vi "S4GUI_002.vi"(7 "Tab ObsEng":enum32{"Obs", "CCD modes", "Eng"}(tab)) -> ()   [LabVIEW 2018] (continued)
            n2632 = call-dynamic "Write PREV_FT.vi"("error in (no error)"=w5539, "PREV_FT"=w5550, "Interface in"=w5546) -> ("error out"=w5542:errorcluster, "Interface out"=w5544:refnum<class "Interface.lvclass">)  [unwired: 7 in]
            n2633 = property on="Exptime ch3" class="DigNum (strict)"("Value"=w5707) -> ()  [unwired: 2 in, 2 out]
            n2634 = call-dynamic "Write PREV_FT.vi"("error in (no error)"=w5643, "PREV_FT"=w5656, "Interface in"=w5645) -> ("error out"=w5649:errorcluster, "Interface out"=w5642:refnum<class "Interface.lvclass">)  [unwired: 7 in]
            n2635 = call-dynamic "Write target cluster.vi"("error in (no error)"=w5591, "target cluster"=w5592, "Channel in"=w5589) -> ("error out"=w5590:errorcluster, "Channel out"=w5588:refnum<class "Channel.lvclass">)  [unwired: 7 in]
            n2636 = call-dynamic "Write target cluster.vi"("error in (no error)"=w5489, "target cluster"=w5488, "Channel in"=w5493) -> ("error out"=w5487:errorcluster, "Channel out"=w5486:refnum<class "Channel.lvclass">)  [unwired: 7 in]
            n2637 = call-dynamic "Write target cluster.vi"("error in (no error)"=w5542, "target cluster"=w5543, "Channel in"=w5537) -> ("error out"=w5538:errorcluster, "Channel out"=w5536:refnum<class "Channel.lvclass">)  [unwired: 7 in]
            n2638 = call-dynamic "Write target cluster.vi"("error in (no error)"=w5649, "target cluster"=w5652, "Channel in"=w5647) -> ("error out"=w5651:errorcluster, "Channel out"=w5650:refnum<class "Channel.lvclass">)  [unwired: 7 in]
            n2639 = Flatten To String(anything=w5592, error in (no error)=w5590) -> (data string=w5625:string, error out=w5626:errorcluster)  [unwired: 2 in, 1 out]
            n2640 = Flatten To String(anything=w5488, error in (no error)=w5487) -> (data string=w5531:string, error out=w5530:errorcluster)  [unwired: 2 in, 1 out]
            n2641 = Flatten To String(anything=w5543, error in (no error)=w5538) -> (data string=w5574:string, error out=w5575:errorcluster)  [unwired: 2 in, 1 out]
            n2642 = Flatten To String(anything=w5652, error in (no error)=w5651) -> (data string=w5684:string, error out=w5683:errorcluster)  [unwired: 2 in, 1 out]
            n2643 = property on="Exptime ch4" class="DigNum (strict)"("Value"=w5707) -> ()  [unwired: 2 in, 2 out]
            n2644 = call "Write flatted cluster.vi"("error in (no error)"=w5626, "flatted cluster"=w5625, "Interface in"=w5587) -> ("error out"=w5628:errorcluster, "Interface out"=w5627:refnum<class "Interface.lvclass">)  [unwired: 7 in]
            n2645 = call "Write flatted cluster.vi"("error in (no error)"=w5530, "flatted cluster"=w5531, "Interface in"=w5495) -> ("error out"=w5528:errorcluster, "Interface out"=w5529:refnum<class "Interface.lvclass">)  [unwired: 7 in]
            n2646 = call "Write flatted cluster.vi"("error in (no error)"=w5575, "flatted cluster"=w5574, "Interface in"=w5544) -> ("error out"=w5577:errorcluster, "Interface out"=w5576:refnum<class "Interface.lvclass">)  [unwired: 7 in]
            n2647 = call "Write flatted cluster.vi"("error in (no error)"=w5683, "flatted cluster"=w5684, "Interface in"=w5642) -> ("error out"=w5681:errorcluster, "Interface out"=w5682:refnum<class "Interface.lvclass">)  [unwired: 7 in]
            n2648 = call-dynamic "Write Interface.vi"("error in (no error)"=w5628, "Interface.lvclass"=w5627, "Channel in"=w5588) -> ("error out"=w5630:errorcluster, "Channel out"=w5631:refnum<class "Channel.lvclass">)  [unwired: 7 in]
            n2649 = call-dynamic "Write Interface.vi"("error in (no error)"=w5528, "Interface.lvclass"=w5529, "Channel in"=w5486) -> ("error out"=w5526:errorcluster, "Channel out"=w5525:refnum<class "Channel.lvclass">)  [unwired: 7 in]
            n2650 = call-dynamic "Write Interface.vi"("error in (no error)"=w5577, "Interface.lvclass"=w5576, "Channel in"=w5536) -> ("error out"=w5579:errorcluster, "Channel out"=w5580:refnum<class "Channel.lvclass">)  [unwired: 7 in]
            n2651 = call-dynamic "Write Interface.vi"("error in (no error)"=w5681, "Interface.lvclass"=w5682, "Channel in"=w5650) -> ("error out"=w5679:errorcluster, "Channel out"=w5678:refnum<class "Channel.lvclass">)  [unwired: 7 in]
            n2652 = call "Write section_name.vi"("error in (no error)"=w5630, "section_name"="CCD_ACS2", "Channel in"=w5631) -> ("error out"=w5629:errorcluster, "Channel out"=w5634:refnum<class "Channel.lvclass">)  [unwired: 7 in]
            n2653 = call "Write section_name.vi"("error in (no error)"=w5526, "section_name"="CCD_ACS4", "Channel in"=w5525) -> ("error out"=w5527:errorcluster, "Channel out"=w5522:refnum<class "Channel.lvclass">)  [unwired: 7 in]
            n2654 = call "Write section_name.vi"("error in (no error)"=w5579, "section_name"="CCD_ACS3", "Channel in"=w5580) -> ("error out"=w5578:errorcluster, "Channel out"=w5583:refnum<class "Channel.lvclass">)  [unwired: 7 in]
            n2655 = call "Write section_name.vi"("error in (no error)"=w5679, "section_name"="CCD_ACS1", "Channel in"=w5678) -> ("error out"=w5680:errorcluster, "Channel out"=w5675:refnum<class "Channel.lvclass">)  [unwired: 7 in]
            n2656 = call-dynamic "save config.vi"("error in (no error)"=w5629, "file config"="lastsaved.cfg", "Channel in"=w5634) -> ("error out"=w5604:errorcluster, "Channel out"=w5605:refnum<class "Channel.lvclass">)  [unwired: 7 in]
            n2657 = call-dynamic "save config.vi"("error in (no error)"=w5527, "file config"="lastsaved.cfg", "Channel in"=w5522) -> ("error out"=w5503:errorcluster, "Channel out"=w5504:refnum<class "Channel.lvclass">)  [unwired: 7 in]
            n2658 = call-dynamic "save config.vi"("error in (no error)"=w5578, "file config"="lastsaved.cfg", "Channel in"=w5583) -> ("error out"=w5552:errorcluster, "Channel out"=w5554:refnum<class "Channel.lvclass">)  [unwired: 7 in]
            n2659 = call-dynamic "save config.vi"("error in (no error)"=w5680, "file config"="lastsaved.cfg", "Channel in"=w5675) -> ("error out"=w5665:errorcluster, "Channel out"=w5666:refnum<class "Channel.lvclass">)  [unwired: 7 in]
            n2660 = local read "Filter2"() -> (w5606:u8)
            n2661 = local read "Filter4"() -> (w5520:u8)
            n2662 = local read "Filter3"() -> (w5570:u8)
            n2663 = local read "Filter1"() -> (w5667:u8)
            n2664 = call-dynamic "Write Filter.vi"("error in (no error)"=w5604, "Filter"=w5606, "Channel in"=w5605) -> ("error out"=w5613:errorcluster, "Channel out"=w5614:refnum<class "Channel.lvclass">)  [unwired: 7 in]
            n2665 = call-dynamic "Write Filter.vi"("error in (no error)"=w5503, "Filter"=w5520, "Channel in"=w5504) -> ("error out"=w5513:errorcluster, "Channel out"=w5512:refnum<class "Channel.lvclass">)  [unwired: 7 in]
            n2666 = call-dynamic "Write Filter.vi"("error in (no error)"=w5552, "Filter"=w5570, "Channel in"=w5554) -> ("error out"=w5563:errorcluster, "Channel out"=w5562:refnum<class "Channel.lvclass">)  [unwired: 7 in]
            n2667 = call-dynamic "Write Filter.vi"("error in (no error)"=w5665, "Filter"=w5667, "Channel in"=w5666) -> ("error out"=w5674:errorcluster, "Channel out"=w5664:refnum<class "Channel.lvclass">)  [unwired: 7 in]
            n2668 = call-dynamic "Read Interface.vi"("error in (no error)"=w5613, "Channel in"=w5614) -> ("error out"=w5611:errorcluster, "Interface.lvclass"=w5616:refnum<class "Interface.lvclass">, "Channel out"=w5615:refnum<class "Channel.lvclass">)  [unwired: 7 in]
            n2669 = call-dynamic "Read Interface.vi"("error in (no error)"=w5513, "Channel in"=w5512) -> ("error out"=w5515:errorcluster, "Interface.lvclass"=w5510:refnum<class "Interface.lvclass">, "Channel out"=w5511:refnum<class "Channel.lvclass">)  [unwired: 7 in]
            n2670 = call-dynamic "Read Interface.vi"("error in (no error)"=w5563, "Channel in"=w5562) -> ("error out"=w5565:errorcluster, "Interface.lvclass"=w5560:refnum<class "Interface.lvclass">, "Channel out"=w5561:refnum<class "Channel.lvclass">)  [unwired: 7 in]
            n2671 = call-dynamic "Read Interface.vi"("error in (no error)"=w5674, "Channel in"=w5664) -> ("error out"=w5672:errorcluster, "Interface.lvclass"=w5663:refnum<class "Interface.lvclass">, "Channel out"=w5657:refnum<class "Channel.lvclass">)  [unwired: 7 in]
            n2672 = call-dynamic "Write Suffix.vi"("error in (no error)"=w5611, "Suffix"=w5689, "Interface in"=w5616) -> ("error out"=w5607:errorcluster, "Interface out"=w5617:refnum<class "Interface.lvclass">)  [unwired: 7 in]
            n2673 = call-dynamic "Write Suffix.vi"("error in (no error)"=w5515, "Suffix"=w5689, "Interface in"=w5510) -> ("error out"=w5519:errorcluster, "Interface out"=w5509:refnum<class "Interface.lvclass">)  [unwired: 7 in]
            n2674 = call-dynamic "Write Suffix.vi"("error in (no error)"=w5565, "Suffix"=w5689, "Interface in"=w5560) -> ("error out"=w5569:errorcluster, "Interface out"=w5559:refnum<class "Interface.lvclass">)  [unwired: 7 in]
            n2675 = call-dynamic "Write Suffix.vi"("error in (no error)"=w5672, "Suffix"=w5689, "Interface in"=w5663) -> ("error out"=w5668:errorcluster, "Interface out"=w5662:refnum<class "Interface.lvclass">)  [unwired: 7 in]
            n2676 = call-dynamic "Write ObsType.vi"("error in (no error)"=w5607, "ObsType"=w5688, "Interface in"=w5617) -> ("error out"=w5608:errorcluster, "Interface out"=w5618:refnum<class "Interface.lvclass">)  [unwired: 7 in]
            n2677 = call-dynamic "Write ObsType.vi"("error in (no error)"=w5519, "ObsType"=w5688, "Interface in"=w5509) -> ("error out"=w5518:errorcluster, "Interface out"=w5508:refnum<class "Interface.lvclass">)  [unwired: 7 in]
            n2678 = call-dynamic "Write ObsType.vi"("error in (no error)"=w5569, "ObsType"=w5688, "Interface in"=w5559) -> ("error out"=w5568:errorcluster, "Interface out"=w5558:refnum<class "Interface.lvclass">)  [unwired: 7 in]
            n2679 = call-dynamic "Write ObsType.vi"("error in (no error)"=w5668, "ObsType"=w5688, "Interface in"=w5662) -> ("error out"=w5669:errorcluster, "Interface out"=w5661:refnum<class "Interface.lvclass">)  [unwired: 7 in]
            n2680 = call-dynamic "Write Object.vi"("error in (no error)"=w5608, "Object"=w5690, "Interface in"=w5618) -> ("error out"=w5609:errorcluster, "Interface out"=w5619:refnum<class "Interface.lvclass">)  [unwired: 7 in]
            n2681 = call-dynamic "Write Object.vi"("error in (no error)"=w5518, "Object"=w5690, "Interface in"=w5508) -> ("error out"=w5517:errorcluster, "Interface out"=w5507:refnum<class "Interface.lvclass">)  [unwired: 7 in]
            n2682 = call-dynamic "Write Object.vi"("error in (no error)"=w5568, "Object"=w5690, "Interface in"=w5558) -> ("error out"=w5567:errorcluster, "Interface out"=w5557:refnum<class "Interface.lvclass">)  [unwired: 7 in]
            n2683 = call-dynamic "Write Object.vi"("error in (no error)"=w5669, "Object"=w5690, "Interface in"=w5661) -> ("error out"=w5670:errorcluster, "Interface out"=w5660:refnum<class "Interface.lvclass">)  [unwired: 7 in]
            n2684 = call-dynamic "Write Comments.vi"("error in (no error)"=w5609, "Comments"=w5691, "Interface in"=w5619) -> ("error out"=w5610:errorcluster, "Interface out"=w5620:refnum<class "Interface.lvclass">)  [unwired: 7 in]
            n2685 = call-dynamic "Write Comments.vi"("error in (no error)"=w5517, "Comments"=w5691, "Interface in"=w5507) -> ("error out"=w5516:errorcluster, "Interface out"=w5506:refnum<class "Interface.lvclass">)  [unwired: 7 in]
            n2686 = call-dynamic "Write Comments.vi"("error in (no error)"=w5567, "Comments"=w5691, "Interface in"=w5557) -> ("error out"=w5566:errorcluster, "Interface out"=w5556:refnum<class "Interface.lvclass">)  [unwired: 7 in]
            n2687 = call-dynamic "Write Comments.vi"("error in (no error)"=w5670, "Comments"=w5691, "Interface in"=w5660) -> ("error out"=w5671:errorcluster, "Interface out"=w5659:refnum<class "Interface.lvclass">)  [unwired: 7 in]
            n2688 = call-dynamic "Write Observer.vi"("error in (no error)"=w5516, "Observer"=w5692, "Interface in"=w5506) -> ("error out"=w5514:errorcluster, "Interface out"=w5505:refnum<class "Interface.lvclass">)  [unwired: 7 in]
            n2689 = call-dynamic "Write Observer.vi"("error in (no error)"=w5566, "Observer"=w5692, "Interface in"=w5556) -> ("error out"=w5564:errorcluster, "Interface out"=w5555:refnum<class "Interface.lvclass">)  [unwired: 7 in]
            n2690 = call-dynamic "Write Observer.vi"("error in (no error)"=w5610, "Observer"=w5692, "Interface in"=w5620) -> ("error out"=w5612:errorcluster, "Interface out"=w5621:refnum<class "Interface.lvclass">)  [unwired: 7 in]
            n2691 = call-dynamic "Write Observer.vi"("error in (no error)"=w5671, "Observer"=w5692, "Interface in"=w5659) -> ("error out"=w5673:errorcluster, "Interface out"=w5658:refnum<class "Interface.lvclass">)  [unwired: 7 in]
            n2692 = call-dynamic "Write Interface.vi"("error in (no error)"=w5514, "Interface.lvclass"=w5505, "Channel in"=w5511) -> ("error out"=w5502:errorcluster, "Channel out"=w5501:refnum<class "Channel.lvclass">)  [unwired: 7 in]
            n2693 = call-dynamic "Write Interface.vi"("error in (no error)"=w5564, "Interface.lvclass"=w5555, "Channel in"=w5561) -> ("error out"=w5551:errorcluster, "Channel out"=w5553:refnum<class "Channel.lvclass">)  [unwired: 7 in]
            n2694 = call-dynamic "Write Interface.vi"("error in (no error)"=w5673, "Interface.lvclass"=w5658, "Channel in"=w5657) -> ("error out"=w5640:errorcluster, "Channel out"=w5641:refnum<class "Channel.lvclass">)  [unwired: 7 in]
            n2695 = call-dynamic "Write Interface.vi"("error in (no error)"=w5612, "Interface.lvclass"=w5621, "Channel in"=w5615) -> ("error out"=w5603:errorcluster, "Channel out"=w5602:refnum<class "Channel.lvclass">)  [unwired: 7 in]
            n2696 = case shown="True" w5637 {
              tunnel: w5641 -> [w5812 w5816]
              tunnel: w5640 -> [w5811 w5815]
              tunnel: [w5812 w5814] -> w5639
              tunnel: [w5811 w5813] -> w5638
              frame False {
              }
              frame True {
                n2697 = call-dynamic "Read State Machine.vi"("error in (no error)"=w5815, "Device in"=w5816) -> ("error out"=w5818:errorcluster, "State Machine.lvclass"=w5821:refnum<class "State Machine.lvclass">, "Device out"=w5833:refnum<class "Channel.lvclass">)  [unwired: 7 in]
                n2698 = call-dynamic "Read ref StatesQueue.vi"("error in (no error)"=w5818, "State Machine in"=w5821) -> ("error out"=w5825:errorcluster, "ref StatesQueue"=w5824:refnum<queue>, "State Machine out"=w5820:refnum<class "State Machine.lvclass">)  [unwired: 7 in]
                n2699 = Flush Queue(queue=w5824, error in (no error)=w5825) -> (queue out=w5826:refnum<queue>, error out=w5830:errorcluster)  [unwired: 1 out]
                n2700 = Enqueue Element(queue=w5826, element=u32 300 ("State"), error in (no error)=w5830) -> (queue out=w5827:refnum<queue>, error out=w5831:errorcluster)  [unwired: 1 in, 1 out]
                n2701 = Enqueue Element(queue=w5827, element=u32 60 ("State"), error in (no error)=w5831) -> (queue out=w5828:refnum<queue>, error out=w5829:errorcluster)  [unwired: 1 in, 1 out]
                n2702 = call-dynamic "Write ref StatesQueue.vi"("error in (no error)"=w5829, "ref StatesQueue"=w5828, "State Machine in"=w5820) -> ("error out"=w5817:errorcluster, "State Machine out"=w5819:refnum<class "State Machine.lvclass">)  [unwired: 7 in]
                n2703 = call-dynamic "Write State.vi"("error in (no error)"=w5817, "State"=0, "State Machine in"=w5819) -> ("error out"=w5835:errorcluster, "State Machine out"=w5832:refnum<class "State Machine.lvclass">)  [unwired: 7 in]
                n2704 = call-dynamic "Write State Machine.vi"("error in (no error)"=w5835, "State Machine.lvclass"=w5832, "Device in"=w5833) -> ("error out"=w5813:errorcluster, "Device out"=w5814:refnum<class "Channel.lvclass">)  [unwired: 7 in]
              }
            }
            n2705 = case shown="True" w5586 {
              tunnel: [w5780 w5804] -> w5636
              tunnel: [w5781 w5803] -> w5635
              tunnel: w5603 -> [w5780 w5798]
              tunnel: w5602 -> [w5781 w5797]
              frame False {
              }
              frame True {
                n2706 = call-dynamic "Read State Machine.vi"("error in (no error)"=w5798, "Device in"=w5797) -> ("error out"=w5783:errorcluster, "State Machine.lvclass"=w5785:refnum<class "State Machine.lvclass">, "Device out"=w5801:refnum<class "Channel.lvclass">)  [unwired: 7 in]
                n2707 = call-dynamic "Read ref StatesQueue.vi"("error in (no error)"=w5783, "State Machine in"=w5785) -> ("error out"=w5790:errorcluster, "ref StatesQueue"=w5789:refnum<queue>, "State Machine out"=w5786:refnum<class "State Machine.lvclass">)  [unwired: 7 in]
                n2708 = Flush Queue(queue=w5789, error in (no error)=w5790) -> (queue out=w5791:refnum<queue>, error out=w5795:errorcluster)  [unwired: 1 out]
                n2709 = Enqueue Element(queue=w5791, element=u32 300 ("State"), error in (no error)=w5795) -> (queue out=w5792:refnum<queue>, error out=w5796:errorcluster)  [unwired: 1 in, 1 out]
                n2710 = Enqueue Element(queue=w5792, element=u32 60 ("State"), error in (no error)=w5796) -> (queue out=w5793:refnum<queue>, error out=w5794:errorcluster)  [unwired: 1 in, 1 out]
                n2711 = call-dynamic "Write ref StatesQueue.vi"("error in (no error)"=w5794, "ref StatesQueue"=w5793, "State Machine in"=w5786) -> ("error out"=w5782:errorcluster, "State Machine out"=w5784:refnum<class "State Machine.lvclass">)  [unwired: 7 in]
                n2712 = call-dynamic "Write State.vi"("error in (no error)"=w5782, "State"=0, "State Machine in"=w5784) -> ("error out"=w5799:errorcluster, "State Machine out"=w5802:refnum<class "State Machine.lvclass">)  [unwired: 7 in]
                n2713 = call-dynamic "Write State Machine.vi"("error in (no error)"=w5799, "State Machine.lvclass"=w5802, "Device in"=w5801) -> ("error out"=w5804:errorcluster, "Device out"=w5803:refnum<class "Channel.lvclass">)  [unwired: 7 in]
              }
            }
            n2714 = case shown="True" w5535 {
              tunnel: [w5750 w5773] -> w5585
              tunnel: [w5749 w5772] -> w5584
              tunnel: w5553 -> [w5749 w5767]
              tunnel: w5551 -> [w5750 w5766]
              frame False {
              }
              frame True {
                n2715 = call-dynamic "Read State Machine.vi"("error in (no error)"=w5766, "Device in"=w5767) -> ("error out"=w5752:errorcluster, "State Machine.lvclass"=w5754:refnum<class "State Machine.lvclass">, "Device out"=w5770:refnum<class "Channel.lvclass">)  [unwired: 7 in]
                n2716 = call-dynamic "Read ref StatesQueue.vi"("error in (no error)"=w5752, "State Machine in"=w5754) -> ("error out"=w5759:errorcluster, "ref StatesQueue"=w5758:refnum<queue>, "State Machine out"=w5755:refnum<class "State Machine.lvclass">)  [unwired: 7 in]
                n2717 = Flush Queue(queue=w5758, error in (no error)=w5759) -> (queue out=w5760:refnum<queue>, error out=w5764:errorcluster)  [unwired: 1 out]
                n2718 = Enqueue Element(queue=w5760, element=u32 300 ("State"), error in (no error)=w5764) -> (queue out=w5761:refnum<queue>, error out=w5765:errorcluster)  [unwired: 1 in, 1 out]
                n2719 = Enqueue Element(queue=w5761, element=u32 60 ("State"), error in (no error)=w5765) -> (queue out=w5762:refnum<queue>, error out=w5763:errorcluster)  [unwired: 1 in, 1 out]
                n2720 = call-dynamic "Write ref StatesQueue.vi"("error in (no error)"=w5763, "ref StatesQueue"=w5762, "State Machine in"=w5755) -> ("error out"=w5751:errorcluster, "State Machine out"=w5753:refnum<class "State Machine.lvclass">)  [unwired: 7 in]
                n2721 = call-dynamic "Write State.vi"("error in (no error)"=w5751, "State"=0, "State Machine in"=w5753) -> ("error out"=w5768:errorcluster, "State Machine out"=w5771:refnum<class "State Machine.lvclass">)  [unwired: 7 in]
                n2722 = call-dynamic "Write State Machine.vi"("error in (no error)"=w5768, "State Machine.lvclass"=w5771, "Device in"=w5770) -> ("error out"=w5773:errorcluster, "Device out"=w5772:refnum<class "Channel.lvclass">)  [unwired: 7 in]
              }
            }
            n2723 = case shown="True" w5484 {
              tunnel: [w5718 w5738] -> w5521
              tunnel: w5502 -> [w5718 w5737]
              tunnel: w5501 -> [w5719 w5736]
              tunnel: [w5719 w5720] -> w5485
              frame False {
              }
              frame True {
                n2724 = call-dynamic "Read State Machine.vi"("error in (no error)"=w5737, "Device in"=w5736) -> ("error out"=w5723:errorcluster, "State Machine.lvclass"=w5724:refnum<class "State Machine.lvclass">, "Device out"=w5740:refnum<class "Channel.lvclass">)  [unwired: 7 in]
                n2725 = call-dynamic "Read ref StatesQueue.vi"("error in (no error)"=w5723, "State Machine in"=w5724) -> ("error out"=w5729:errorcluster, "ref StatesQueue"=w5728:refnum<queue>, "State Machine out"=w5725:refnum<class "State Machine.lvclass">)  [unwired: 7 in]
                n2726 = Flush Queue(queue=w5728, error in (no error)=w5729) -> (queue out=w5730:refnum<queue>, error out=w5734:errorcluster)  [unwired: 1 out]
                n2727 = Enqueue Element(queue=w5730, element=u32 300 ("State"), error in (no error)=w5734) -> (queue out=w5731:refnum<queue>, error out=w5735:errorcluster)  [unwired: 1 in, 1 out]
                n2728 = Enqueue Element(queue=w5731, element=u32 60 ("State"), error in (no error)=w5735) -> (queue out=w5732:refnum<queue>, error out=w5733:errorcluster)  [unwired: 1 in, 1 out]
                n2729 = call-dynamic "Write ref StatesQueue.vi"("error in (no error)"=w5733, "ref StatesQueue"=w5732, "State Machine in"=w5725) -> ("error out"=w5722:errorcluster, "State Machine out"=w5721:refnum<class "State Machine.lvclass">)  [unwired: 7 in]
                n2730 = call-dynamic "Write State.vi"("error in (no error)"=w5722, "State"=0, "State Machine in"=w5721) -> ("error out"=w5742:errorcluster, "State Machine out"=w5739:refnum<class "State Machine.lvclass">)  [unwired: 7 in]
                n2731 = call-dynamic "Write State Machine.vi"("error in (no error)"=w5742, "State Machine.lvclass"=w5739, "Device in"=w5740) -> ("error out"=w5738:errorcluster, "Device out"=w5720:refnum<class "Channel.lvclass">)  [unwired: 7 in]
              }
            }
            n2732 = call-dynamic "Write Channel.vi"("error in (no error)"=w5636, "Channel.lvclass"=w5635, "Acquisition in"=w5622) -> ("error out"=w5714:errorcluster, "Acquisition out"=w5715:refnum<class "Acquisition.lvclass">)  [unwired: 7 in]
            n2733 = call-dynamic "Write Channel.vi"("error in (no error)"=w5638, "Channel.lvclass"=w5639, "Acquisition in"=w5687) -> ("error out"=w5716:errorcluster, "Acquisition out"=w5717:refnum<class "Acquisition.lvclass">)  [unwired: 7 in]
            n2734 = call-dynamic "Write Channel.vi"("error in (no error)"=w5585, "Channel.lvclass"=w5584, "Acquisition in"=w5571) -> ("error out"=w5712:errorcluster, "Acquisition out"=w5713:refnum<class "Acquisition.lvclass">)  [unwired: 7 in]
            n2735 = call-dynamic "Write Channel.vi"("error in (no error)"=w5521, "Channel.lvclass"=w5485, "Acquisition in"=w5534) -> ("error out"=w5710:errorcluster, "Acquisition out"=w5711:refnum<class "Acquisition.lvclass">)  [unwired: 7 in]
          }
          frame "DARK" {
            # "nome do arquivo .cfg"
            # "seção no arquivo .cfg"
            # "closed"
            # "nome do arquivo .cfg"
            # "seção no arquivo .cfg"
            # "closed"
            # "nome do arquivo .cfg"
            # "seção no arquivo .cfg"
            # "closed"
            # "nome do arquivo .cfg"
            # "seção no arquivo .cfg"
            # "closed"
            # "DARK: Shutter automatically closed and restore FRAME_TRANSFER."
            n2736 = call "Read connection.vi"("error in (no error)"=w6063, "Server in"=w6064) -> ("error out"=w6069:errorcluster, "connection"=w5842:bool, "Server out"=w6070:refnum<class "Acquisition.lvclass">)  [unwired: 7 in]
            n2737 = call "Read connection.vi"("error in (no error)"=w6067, "Server in"=w6068) -> ("error out"=w6073:errorcluster, "connection"=w5844:bool, "Server out"=w6074:refnum<class "Acquisition.lvclass">)  [unwired: 7 in]
            n2738 = call "Read connection.vi"("error in (no error)"=w6065, "Server in"=w6066) -> ("error out"=w6071:errorcluster, "connection"=w5843:bool, "Server out"=w6072:refnum<class "Acquisition.lvclass">)  [unwired: 7 in]
            n2739 = call "Read connection.vi"("error in (no error)"=w6077, "Server in"=w6078) -> ("error out"=w6075:errorcluster, "connection"=w5845:bool, "Server out"=w6076:refnum<class "Acquisition.lvclass">)  [unwired: 7 in]
            n2740 = call-dynamic "Read Channel.vi"("error in (no error)"=w6069, "Acquisition in"=w6070) -> ("error out"=w5896:errorcluster, "Channel.lvclass"=w5897:refnum<class "Channel.lvclass">, "Acquisition out"=w5898:refnum<class "Acquisition.lvclass">)  [unwired: 7 in]
            n2741 = call-dynamic "Read Channel.vi"("error in (no error)"=w6073, "Acquisition in"=w6074) -> ("error out"=w5991:errorcluster, "Channel.lvclass"=w5990:refnum<class "Channel.lvclass">, "Acquisition out"=w5989:refnum<class "Acquisition.lvclass">)  [unwired: 7 in]
            n2742 = call-dynamic "Read Channel.vi"("error in (no error)"=w6075, "Acquisition in"=w6076) -> ("error out"=w6055:errorcluster, "Channel.lvclass"=w6056:refnum<class "Channel.lvclass">, "Acquisition out"=w6057:refnum<class "Acquisition.lvclass">)  [unwired: 7 in]
            n2743 = call-dynamic "Read Channel.vi"("error in (no error)"=w6071, "Acquisition in"=w6072) -> ("error out"=w5938:errorcluster, "Channel.lvclass"=w5937:refnum<class "Channel.lvclass">, "Acquisition out"=w5936:refnum<class "Acquisition.lvclass">)  [unwired: 7 in]
            n2744 = call-dynamic "Read Interface.vi"("error in (no error)"=w5896, "Channel in"=w5897) -> ("error out"=w5859:errorcluster, "Interface.lvclass"=w5858:refnum<class "Interface.lvclass">, "Channel out"=w5854:refnum<class "Channel.lvclass">)  [unwired: 7 in]
            n2745 = call-dynamic "Read Interface.vi"("error in (no error)"=w5991, "Channel in"=w5990) -> ("error out"=w5965:errorcluster, "Interface.lvclass"=w5964:refnum<class "Interface.lvclass">, "Channel out"=w5960:refnum<class "Channel.lvclass">)  [unwired: 7 in]
            n2746 = call-dynamic "Read Interface.vi"("error in (no error)"=w6055, "Channel in"=w6056) -> ("error out"=w6017:errorcluster, "Interface.lvclass"=w6018:refnum<class "Interface.lvclass">, "Channel out"=w6013:refnum<class "Channel.lvclass">)  [unwired: 7 in]
            n2747 = call-dynamic "Read Interface.vi"("error in (no error)"=w5938, "Channel in"=w5937) -> ("error out"=w5910:errorcluster, "Interface.lvclass"=w5912:refnum<class "Interface.lvclass">, "Channel out"=w5907:refnum<class "Channel.lvclass">)  [unwired: 7 in]
            n2748 = call-dynamic "Read restoreExpTime.vi"("error in (no error)"=w5965, "Interface in"=w5964) -> ("error out"=w5962:errorcluster, "restoreExpTime"=w5961:bool, "Interface out"=w5963:refnum<class "Interface.lvclass">)  [unwired: 7 in]
            n2749 = call-dynamic "Read restoreExpTime.vi"("error in (no error)"=w6017, "Interface in"=w6018) -> ("error out"=w6015:errorcluster, "restoreExpTime"=w6014:bool, "Interface out"=w6016:refnum<class "Interface.lvclass">)  [unwired: 7 in]
            n2750 = call-dynamic "Read restoreExpTime.vi"("error in (no error)"=w5859, "Interface in"=w5858) -> ("error out"=w5856:errorcluster, "restoreExpTime"=w5855:bool, "Interface out"=w5857:refnum<class "Interface.lvclass">)  [unwired: 7 in]
            n2751 = call-dynamic "Read restoreExpTime.vi"("error in (no error)"=w5910, "Interface in"=w5912) -> ("error out"=w5909:errorcluster, "restoreExpTime"=w5908:bool, "Interface out"=w5911:refnum<class "Interface.lvclass">)  [unwired: 7 in]
            n2752 = case shown="True" w5961 {
              tunnel: w5963 -> [w6208 w6213]
              tunnel: [w6208 w6216] -> w5967
              tunnel: w5962 -> [w6207 w6211]
              tunnel: [w6207 w6215] -> w5966
              frame False {
              }
              frame True {
                n2753 = call-dynamic "Write restoreExpTime.vi"("error in (no error)"=w6211, "restoreExpTime"=FALSE, "Interface in"=w6213) -> ("error out"=w6210:errorcluster, "Interface out"=w6212:refnum<class "Interface.lvclass">)  [unwired: 7 in]
                n2754 = call-dynamic "Read prev ExpTime.vi"("error in (no error)"=w6210, "Interface in"=w6212) -> ("error out"=w6215:errorcluster, "prev ExpTime"=w6214:dbl, "Interface out"=w6216:refnum<class "Interface.lvclass">)  [unwired: 7 in]
                n2755 = property on="Exptime ch2" class="DigNum (strict)"("Value"=w6214) -> ()  [unwired: 2 in, 2 out]
              }
            }
            n2756 = case shown="True" w6014 {
              tunnel: [w6218 w6226] -> w6020
              tunnel: [w6217 w6225] -> w6019
              tunnel: w6016 -> [w6218 w6223]
              tunnel: w6015 -> [w6217 w6221]
              frame False {
              }
              frame True {
                n2757 = call-dynamic "Write restoreExpTime.vi"("error in (no error)"=w6221, "restoreExpTime"=FALSE, "Interface in"=w6223) -> ("error out"=w6220:errorcluster, "Interface out"=w6222:refnum<class "Interface.lvclass">)  [unwired: 7 in]
                n2758 = call-dynamic "Read prev ExpTime.vi"("error in (no error)"=w6220, "Interface in"=w6222) -> ("error out"=w6225:errorcluster, "prev ExpTime"=w6224:dbl, "Interface out"=w6226:refnum<class "Interface.lvclass">)  [unwired: 7 in]
                n2759 = property on="Exptime ch1" class="DigNum (strict)"("Value"=w6224) -> ()  [unwired: 2 in, 2 out]
              }
            }
            n2760 = case shown="True" w5855 {
              tunnel: w5857 -> [w6188 w6193]
              tunnel: w5856 -> [w6187 w6191]
              tunnel: [w6187 w6196] -> w5861
              tunnel: [w6188 w6195] -> w5860
              frame False {
              }
              frame True {
                n2761 = call-dynamic "Write restoreExpTime.vi"("error in (no error)"=w6191, "restoreExpTime"=FALSE, "Interface in"=w6193) -> ("error out"=w6189:errorcluster, "Interface out"=w6192:refnum<class "Interface.lvclass">)  [unwired: 7 in]
                n2762 = call-dynamic "Read prev ExpTime.vi"("error in (no error)"=w6189, "Interface in"=w6192) -> ("error out"=w6196:errorcluster, "prev ExpTime"=w6194:dbl, "Interface out"=w6195:refnum<class "Interface.lvclass">)  [unwired: 7 in]
                n2763 = property on="Exptime ch4" class="DigNum (strict)"("Value"=w6194) -> ()  [unwired: 2 in, 2 out]
              }
            }
            n2764 = case shown="True" w5908 {
              tunnel: w5911 -> [w6198 w6203]
              tunnel: [w6198 w6206] -> w5914
              tunnel: w5909 -> [w6197 w6202]
              tunnel: [w6197 w6205] -> w5913
              frame False {
              }
              frame True {
                n2765 = call-dynamic "Write restoreExpTime.vi"("error in (no error)"=w6202, "restoreExpTime"=FALSE, "Interface in"=w6203) -> ("error out"=w6199:errorcluster, "Interface out"=w6200:refnum<class "Interface.lvclass">)  [unwired: 7 in]
                n2766 = call-dynamic "Read prev ExpTime.vi"("error in (no error)"=w6199, "Interface in"=w6200) -> ("error out"=w6205:errorcluster, "prev ExpTime"=w6204:dbl, "Interface out"=w6206:refnum<class "Interface.lvclass">)  [unwired: 7 in]
                n2767 = property on="Exptime ch3" class="DigNum (strict)"("Value"=w6204) -> ()  [unwired: 2 in, 2 out]
              }
            }
            n2768 = call-dynamic "Read PREV_FT.vi"("error in (no error)"=w5861, "Interface in"=w5860) -> ("error out"=w5853:errorcluster, "PREV_FT"=w5862:bool, "Interface out"=w5851:refnum<class "Interface.lvclass">)  [unwired: 7 in]
            n2769 = call-dynamic "Read PREV_FT.vi"("error in (no error)"=w5966, "Interface in"=w5967) -> ("error out"=w5959:errorcluster, "PREV_FT"=w5968:bool, "Interface out"=w5957:refnum<class "Interface.lvclass">)  [unwired: 7 in]
            n2770 = call-dynamic "Read PREV_FT.vi"("error in (no error)"=w6019, "Interface in"=w6020) -> ("error out"=w6010:errorcluster, "PREV_FT"=w6021:bool, "Interface out"=w6005:refnum<class "Interface.lvclass">)  [unwired: 7 in]
            n2771 = call-dynamic "Read PREV_FT.vi"("error in (no error)"=w5913, "Interface in"=w5914) -> ("error out"=w5906:errorcluster, "PREV_FT"=w5915:bool, "Interface out"=w5904:refnum<class "Interface.lvclass">)  [unwired: 7 in]
            n2772 = call-dynamic "Read target cluster.vi"("error in (no error)"=w5853, "Channel in"=w5854) -> ("error out"=w5848:errorcluster, "target cluster"=w5852:T31, "Channel out"=w5850:refnum<class "Channel.lvclass">)  [unwired: 7 in]
            n2773 = Bundle By Name(cluster=w5852, "SHUTTER_MODE"=u8 2, "FRAME_TRANSFER"=w5862) -> (w5849:T31)
            n2774 = call-dynamic "Read target cluster.vi"("error in (no error)"=w5959, "Channel in"=w5960) -> ("error out"=w5954:errorcluster, "target cluster"=w5958:T31, "Channel out"=w5956:refnum<class "Channel.lvclass">)  [unwired: 7 in]
            n2775 = Bundle By Name(cluster=w5958, "SHUTTER_MODE"=u8 2, "FRAME_TRANSFER"=w5968) -> (w5955:T31)
            n2776 = call-dynamic "Read target cluster.vi"("error in (no error)"=w5906, "Channel in"=w5907) -> ("error out"=w5901:errorcluster, "target cluster"=w5905:T31, "Channel out"=w5903:refnum<class "Channel.lvclass">)  [unwired: 7 in]
            n2777 = Bundle By Name(cluster=w5905, "SHUTTER_MODE"=u8 2, "FRAME_TRANSFER"=w5915) -> (w5902:T31)
            n2778 = call-dynamic "Read target cluster.vi"("error in (no error)"=w6010, "Channel in"=w6013) -> ("error out"=w6009:errorcluster, "target cluster"=w6007:T31, "Channel out"=w6012:refnum<class "Channel.lvclass">)  [unwired: 7 in]
            n2779 = Bundle By Name(cluster=w6007, "SHUTTER_MODE"=u8 2, "FRAME_TRANSFER"=w6021) -> (w6006:T31)
            n2780 = call-dynamic "Write target cluster.vi"("error in (no error)"=w6009, "target cluster"=w6006, "Channel in"=w6012) -> ("error out"=w6008:errorcluster, "Channel out"=w6011:refnum<class "Channel.lvclass">)  [unwired: 7 in]
            n2781 = call-dynamic "Write target cluster.vi"("error in (no error)"=w5848, "target cluster"=w5849, "Channel in"=w5850) -> ("error out"=w5847:errorcluster, "Channel out"=w5846:refnum<class "Channel.lvclass">)  [unwired: 7 in]
            n2782 = call-dynamic "Write target cluster.vi"("error in (no error)"=w5954, "target cluster"=w5955, "Channel in"=w5956) -> ("error out"=w5953:errorcluster, "Channel out"=w5952:refnum<class "Channel.lvclass">)  [unwired: 7 in]
            n2783 = call-dynamic "Write target cluster.vi"("error in (no error)"=w5901, "target cluster"=w5902, "Channel in"=w5903) -> ("error out"=w5900:errorcluster, "Channel out"=w5899:refnum<class "Channel.lvclass">)  [unwired: 7 in]
            n2784 = Flatten To String(anything=w6006, error in (no error)=w6008) -> (data string=w6054:string, error out=w6053:errorcluster)  [unwired: 2 in, 1 out]
            n2785 = Flatten To String(anything=w5849, error in (no error)=w5847) -> (data string=w5895:string, error out=w5894:errorcluster)  [unwired: 2 in, 1 out]
            n2786 = Flatten To String(anything=w5955, error in (no error)=w5953) -> (data string=w5992:string, error out=w5993:errorcluster)  [unwired: 2 in, 1 out]
            n2787 = Flatten To String(anything=w5902, error in (no error)=w5900) -> (data string=w5939:string, error out=w5940:errorcluster)  [unwired: 2 in, 1 out]
            n2788 = call "Write flatted cluster.vi"("error in (no error)"=w6053, "flatted cluster"=w6054, "Interface in"=w6005) -> ("error out"=w6050:errorcluster, "Interface out"=w6051:refnum<class "Interface.lvclass">)  [unwired: 7 in]
            n2789 = call "Write flatted cluster.vi"("error in (no error)"=w5894, "flatted cluster"=w5895, "Interface in"=w5851) -> ("error out"=w5891:errorcluster, "Interface out"=w5892:refnum<class "Interface.lvclass">)  [unwired: 7 in]
            n2790 = call "Write flatted cluster.vi"("error in (no error)"=w5993, "flatted cluster"=w5992, "Interface in"=w5957) -> ("error out"=w5996:errorcluster, "Interface out"=w5995:refnum<class "Interface.lvclass">)  [unwired: 7 in]
            n2791 = call "Write flatted cluster.vi"("error in (no error)"=w5940, "flatted cluster"=w5939, "Interface in"=w5904) -> ("error out"=w5943:errorcluster, "Interface out"=w5942:refnum<class "Interface.lvclass">)  [unwired: 7 in]
            n2792 = call-dynamic "Write Interface.vi"("error in (no error)"=w6050, "Interface.lvclass"=w6051, "Channel in"=w6011) -> ("error out"=w6048:errorcluster, "Channel out"=w6047:refnum<class "Channel.lvclass">)  [unwired: 7 in]
            n2793 = call-dynamic "Write Interface.vi"("error in (no error)"=w5891, "Interface.lvclass"=w5892, "Channel in"=w5846) -> ("error out"=w5889:errorcluster, "Channel out"=w5888:refnum<class "Channel.lvclass">)  [unwired: 7 in]
            n2794 = call-dynamic "Write Interface.vi"("error in (no error)"=w5996, "Interface.lvclass"=w5995, "Channel in"=w5952) -> ("error out"=w5998:errorcluster, "Channel out"=w5999:refnum<class "Channel.lvclass">)  [unwired: 7 in]
            n2795 = call-dynamic "Write Interface.vi"("error in (no error)"=w5943, "Interface.lvclass"=w5942, "Channel in"=w5899) -> ("error out"=w5945:errorcluster, "Channel out"=w5946:refnum<class "Channel.lvclass">)  [unwired: 7 in]
            n2796 = call "Write section_name.vi"("error in (no error)"=w6048, "section_name"="CCD_ACS1", "Channel in"=w6047) -> ("error out"=w6049:errorcluster, "Channel out"=w6044:refnum<class "Channel.lvclass">)  [unwired: 7 in]
            n2797 = call "Write section_name.vi"("error in (no error)"=w5889, "section_name"="CCD_ACS4", "Channel in"=w5888) -> ("error out"=w5890:errorcluster, "Channel out"=w5885:refnum<class "Channel.lvclass">)  [unwired: 7 in]
            n2798 = call "Write section_name.vi"("error in (no error)"=w5998, "section_name"="CCD_ACS2", "Channel in"=w5999) -> ("error out"=w5997:errorcluster, "Channel out"=w6002:refnum<class "Channel.lvclass">)  [unwired: 7 in]
            n2799 = call "Write section_name.vi"("error in (no error)"=w5945, "section_name"="CCD_ACS3", "Channel in"=w5946) -> ("error out"=w5944:errorcluster, "Channel out"=w5949:refnum<class "Channel.lvclass">)  [unwired: 7 in]
            n2800 = call-dynamic "save config.vi"("error in (no error)"=w6049, "file config"="lastsaved.cfg", "Channel in"=w6044) -> ("error out"=w6024:errorcluster, "Channel out"=w6025:refnum<class "Channel.lvclass">)  [unwired: 7 in]
            n2801 = call-dynamic "save config.vi"("error in (no error)"=w5890, "file config"="lastsaved.cfg", "Channel in"=w5885) -> ("error out"=w5865:errorcluster, "Channel out"=w5866:refnum<class "Channel.lvclass">)  [unwired: 7 in]
            n2802 = call-dynamic "save config.vi"("error in (no error)"=w5997, "file config"="lastsaved.cfg", "Channel in"=w6002) -> ("error out"=w5971:errorcluster, "Channel out"=w5972:refnum<class "Channel.lvclass">)  [unwired: 7 in]
            n2803 = call-dynamic "save config.vi"("error in (no error)"=w5944, "file config"="lastsaved.cfg", "Channel in"=w5949) -> ("error out"=w5918:errorcluster, "Channel out"=w5919:refnum<class "Channel.lvclass">)  [unwired: 7 in]
            n2804 = local read "Filter1"() -> (w6026:u8)
            n2805 = local read "Filter2"() -> (w5973:u8)
            n2806 = local read "Filter4"() -> (w5867:u8)
            n2807 = local read "Filter3"() -> (w5920:u8)
            n2808 = call-dynamic "Write Filter.vi"("error in (no error)"=w6024, "Filter"=w6026, "Channel in"=w6025) -> ("error out"=w6033:errorcluster, "Channel out"=w6034:refnum<class "Channel.lvclass">)  [unwired: 7 in]
            n2809 = call-dynamic "Write Filter.vi"("error in (no error)"=w5918, "Filter"=w5920, "Channel in"=w5919) -> ("error out"=w5927:errorcluster, "Channel out"=w5928:refnum<class "Channel.lvclass">)  [unwired: 7 in]
            n2810 = call-dynamic "Write Filter.vi"("error in (no error)"=w5971, "Filter"=w5973, "Channel in"=w5972) -> ("error out"=w5980:errorcluster, "Channel out"=w5981:refnum<class "Channel.lvclass">)  [unwired: 7 in]
            n2811 = call-dynamic "Write Filter.vi"("error in (no error)"=w5865, "Filter"=w5867, "Channel in"=w5866) -> ("error out"=w5874:errorcluster, "Channel out"=w5875:refnum<class "Channel.lvclass">)  [unwired: 7 in]
            n2812 = call-dynamic "Read Interface.vi"("error in (no error)"=w5980, "Channel in"=w5981) -> ("error out"=w5978:errorcluster, "Interface.lvclass"=w5983:refnum<class "Interface.lvclass">, "Channel out"=w5982:refnum<class "Channel.lvclass">)  [unwired: 7 in]
            n2813 = call-dynamic "Read Interface.vi"("error in (no error)"=w5927, "Channel in"=w5928) -> ("error out"=w5925:errorcluster, "Interface.lvclass"=w5930:refnum<class "Interface.lvclass">, "Channel out"=w5929:refnum<class "Channel.lvclass">)  [unwired: 7 in]
            n2814 = call-dynamic "Read Interface.vi"("error in (no error)"=w6033, "Channel in"=w6034) -> ("error out"=w6031:errorcluster, "Interface.lvclass"=w6036:refnum<class "Interface.lvclass">, "Channel out"=w6035:refnum<class "Channel.lvclass">)  [unwired: 7 in]
            n2815 = call-dynamic "Read Interface.vi"("error in (no error)"=w5874, "Channel in"=w5875) -> ("error out"=w5872:errorcluster, "Interface.lvclass"=w5877:refnum<class "Interface.lvclass">, "Channel out"=w5876:refnum<class "Channel.lvclass">)  [unwired: 7 in]
            n2816 = call-dynamic "Write Suffix.vi"("error in (no error)"=w6031, "Suffix"=w6059, "Interface in"=w6036) -> ("error out"=w6027:errorcluster, "Interface out"=w6037:refnum<class "Interface.lvclass">)  [unwired: 7 in]
            n2817 = call-dynamic "Write Suffix.vi"("error in (no error)"=w5978, "Suffix"=w6059, "Interface in"=w5983) -> ("error out"=w5974:errorcluster, "Interface out"=w5984:refnum<class "Interface.lvclass">)  [unwired: 7 in]
            n2818 = call-dynamic "Write Suffix.vi"("error in (no error)"=w5925, "Suffix"=w6059, "Interface in"=w5930) -> ("error out"=w5921:errorcluster, "Interface out"=w5931:refnum<class "Interface.lvclass">)  [unwired: 7 in]
            n2819 = call-dynamic "Write Suffix.vi"("error in (no error)"=w5872, "Suffix"=w6059, "Interface in"=w5877) -> ("error out"=w5868:errorcluster, "Interface out"=w5878:refnum<class "Interface.lvclass">)  [unwired: 7 in]
            n2820 = call-dynamic "Write ObsType.vi"("error in (no error)"=w5974, "ObsType"=w6058, "Interface in"=w5984) -> ("error out"=w5975:errorcluster, "Interface out"=w5985:refnum<class "Interface.lvclass">)  [unwired: 7 in]
            n2821 = call-dynamic "Write ObsType.vi"("error in (no error)"=w5921, "ObsType"=w6058, "Interface in"=w5931) -> ("error out"=w5922:errorcluster, "Interface out"=w5932:refnum<class "Interface.lvclass">)  [unwired: 7 in]
            n2822 = call-dynamic "Write ObsType.vi"("error in (no error)"=w6027, "ObsType"=w6058, "Interface in"=w6037) -> ("error out"=w6028:errorcluster, "Interface out"=w6038:refnum<class "Interface.lvclass">)  [unwired: 7 in]
            n2823 = call-dynamic "Write ObsType.vi"("error in (no error)"=w5868, "ObsType"=w6058, "Interface in"=w5878) -> ("error out"=w5869:errorcluster, "Interface out"=w5879:refnum<class "Interface.lvclass">)  [unwired: 7 in]
            n2824 = call-dynamic "Write Object.vi"("error in (no error)"=w5975, "Object"=w6062, "Interface in"=w5985) -> ("error out"=w5976:errorcluster, "Interface out"=w5986:refnum<class "Interface.lvclass">)  [unwired: 7 in]
            n2825 = call-dynamic "Write Object.vi"("error in (no error)"=w5922, "Object"=w6062, "Interface in"=w5932) -> ("error out"=w5923:errorcluster, "Interface out"=w5933:refnum<class "Interface.lvclass">)  [unwired: 7 in]
            n2826 = call-dynamic "Write Object.vi"("error in (no error)"=w6028, "Object"=w6062, "Interface in"=w6038) -> ("error out"=w6029:errorcluster, "Interface out"=w6039:refnum<class "Interface.lvclass">)  [unwired: 7 in]
            n2827 = call-dynamic "Write Object.vi"("error in (no error)"=w5869, "Object"=w6062, "Interface in"=w5879) -> ("error out"=w5870:errorcluster, "Interface out"=w5880:refnum<class "Interface.lvclass">)  [unwired: 7 in]
            n2828 = call-dynamic "Write Comments.vi"("error in (no error)"=w5976, "Comments"=w6061, "Interface in"=w5986) -> ("error out"=w5977:errorcluster, "Interface out"=w5987:refnum<class "Interface.lvclass">)  [unwired: 7 in]
            n2829 = call-dynamic "Write Comments.vi"("error in (no error)"=w5923, "Comments"=w6061, "Interface in"=w5933) -> ("error out"=w5924:errorcluster, "Interface out"=w5934:refnum<class "Interface.lvclass">)  [unwired: 7 in]
            n2830 = call-dynamic "Write Comments.vi"("error in (no error)"=w6029, "Comments"=w6061, "Interface in"=w6039) -> ("error out"=w6030:errorcluster, "Interface out"=w6040:refnum<class "Interface.lvclass">)  [unwired: 7 in]
            n2831 = call-dynamic "Write Comments.vi"("error in (no error)"=w5870, "Comments"=w6061, "Interface in"=w5880) -> ("error out"=w5871:errorcluster, "Interface out"=w5881:refnum<class "Interface.lvclass">)  [unwired: 7 in]
            n2832 = call-dynamic "Write Observer.vi"("error in (no error)"=w5977, "Observer"=w6060, "Interface in"=w5987) -> ("error out"=w5979:errorcluster, "Interface out"=w5988:refnum<class "Interface.lvclass">)  [unwired: 7 in]
            n2833 = call-dynamic "Write Observer.vi"("error in (no error)"=w5924, "Observer"=w6060, "Interface in"=w5934) -> ("error out"=w5926:errorcluster, "Interface out"=w5935:refnum<class "Interface.lvclass">)  [unwired: 7 in]
            n2834 = call-dynamic "Write Observer.vi"("error in (no error)"=w6030, "Observer"=w6060, "Interface in"=w6040) -> ("error out"=w6032:errorcluster, "Interface out"=w6041:refnum<class "Interface.lvclass">)  [unwired: 7 in]
            n2835 = call-dynamic "Write Observer.vi"("error in (no error)"=w5871, "Observer"=w6060, "Interface in"=w5881) -> ("error out"=w5873:errorcluster, "Interface out"=w5882:refnum<class "Interface.lvclass">)  [unwired: 7 in]
            n2836 = call-dynamic "Write Interface.vi"("error in (no error)"=w5979, "Interface.lvclass"=w5988, "Channel in"=w5982) -> ("error out"=w5969:errorcluster, "Channel out"=w5970:refnum<class "Channel.lvclass">)  [unwired: 7 in]
            n2837 = call-dynamic "Write Interface.vi"("error in (no error)"=w5926, "Interface.lvclass"=w5935, "Channel in"=w5929) -> ("error out"=w5916:errorcluster, "Channel out"=w5917:refnum<class "Channel.lvclass">)  [unwired: 7 in]
            n2838 = call-dynamic "Write Interface.vi"("error in (no error)"=w6032, "Interface.lvclass"=w6041, "Channel in"=w6035) -> ("error out"=w6022:errorcluster, "Channel out"=w6023:refnum<class "Channel.lvclass">)  [unwired: 7 in]
            n2839 = call-dynamic "Write Interface.vi"("error in (no error)"=w5873, "Interface.lvclass"=w5882, "Channel in"=w5876) -> ("error out"=w5863:errorcluster, "Channel out"=w5864:refnum<class "Channel.lvclass">)  [unwired: 7 in]
            n2840 = case shown="True" w5845 {
              tunnel: [w6163 w6182] -> w6043
              tunnel: [w6162 w6181] -> w6042
              tunnel: w6023 -> [w6163 w6180]
              tunnel: w6022 -> [w6162 w6179]
              frame False {
              }
              frame True {
                # "command WRITE_SETUP"
                # "command SET SUFFIX"
                n2841 = call-dynamic "Read State Machine.vi"("error in (no error)"=w6179, "Device in"=w6180) -> ("error out"=w6167:errorcluster, "State Machine.lvclass"=w6169:refnum<class "State Machine.lvclass">, "Device out"=w6184:refnum<class "Channel.lvclass">)  [unwired: 7 in]
                n2842 = call-dynamic "Read ref StatesQueue.vi"("error in (no error)"=w6167, "State Machine in"=w6169) -> ("error out"=w6177:errorcluster, "ref StatesQueue"=w6165:refnum<queue>, "State Machine out"=w6178:refnum<class "State Machine.lvclass">)  [unwired: 7 in]
                n2843 = Flush Queue(queue=w6165, error in (no error)=w6177) -> (queue out=w6164:refnum<queue>, error out=w6173:errorcluster)  [unwired: 1 out]
                n2844 = Enqueue Element(queue=w6164, element=u32 300 ("State"), error in (no error)=w6173) -> (queue out=w6176:refnum<queue>, error out=w6172:errorcluster)  [unwired: 1 in, 1 out]
                n2845 = Enqueue Element(queue=w6176, element=u32 60 ("State"), error in (no error)=w6172) -> (queue out=w6175:refnum<queue>, error out=w6174:errorcluster)  [unwired: 1 in, 1 out]
                n2846 = call-dynamic "Write ref StatesQueue.vi"("error in (no error)"=w6174, "ref StatesQueue"=w6175, "State Machine in"=w6178) -> ("error out"=w6166:errorcluster, "State Machine out"=w6168:refnum<class "State Machine.lvclass">)  [unwired: 7 in]
                n2847 = call-dynamic "Write State.vi"("error in (no error)"=w6166, "State"=0, "State Machine in"=w6168) -> ("error out"=w6186:errorcluster, "State Machine out"=w6183:refnum<class "State Machine.lvclass">)  [unwired: 7 in]
                n2848 = call-dynamic "Write State Machine.vi"("error in (no error)"=w6186, "State Machine.lvclass"=w6183, "Device in"=w6184) -> ("error out"=w6181:errorcluster, "Device out"=w6182:refnum<class "Channel.lvclass">)  [unwired: 7 in]
              }
            }
            n2849 = case shown="True" w5844 {
              tunnel: [w6137 w6161] -> w6004
              tunnel: [w6138 w6160] -> w6003
              tunnel: w5970 -> [w6138 w6155]
              tunnel: w5969 -> [w6137 w6154]
              frame False {
              }
              frame True {
                # "command WRITE_SETUP"
                # "command SET SUFFIX"
                n2850 = call-dynamic "Read State Machine.vi"("error in (no error)"=w6154, "Device in"=w6155) -> ("error out"=w6143:errorcluster, "State Machine.lvclass"=w6144:refnum<class "State Machine.lvclass">, "Device out"=w6158:refnum<class "Channel.lvclass">)  [unwired: 7 in]
                n2851 = call-dynamic "Read ref StatesQueue.vi"("error in (no error)"=w6143, "State Machine in"=w6144) -> ("error out"=w6152:errorcluster, "ref StatesQueue"=w6142:refnum<queue>, "State Machine out"=w6153:refnum<class "State Machine.lvclass">)  [unwired: 7 in]
                n2852 = Flush Queue(queue=w6142, error in (no error)=w6152) -> (queue out=w6141:refnum<queue>, error out=w6148:errorcluster)  [unwired: 1 out]
                n2853 = Enqueue Element(queue=w6141, element=u32 300 ("State"), error in (no error)=w6148) -> (queue out=w6151:refnum<queue>, error out=w6147:errorcluster)  [unwired: 1 in, 1 out]
                n2854 = Enqueue Element(queue=w6151, element=u32 60 ("State"), error in (no error)=w6147) -> (queue out=w6150:refnum<queue>, error out=w6149:errorcluster)  [unwired: 1 in, 1 out]
                n2855 = call-dynamic "Write ref StatesQueue.vi"("error in (no error)"=w6149, "ref StatesQueue"=w6150, "State Machine in"=w6153) -> ("error out"=w6139:errorcluster, "State Machine out"=w6140:refnum<class "State Machine.lvclass">)  [unwired: 7 in]
                n2856 = call-dynamic "Write State.vi"("error in (no error)"=w6139, "State"=0, "State Machine in"=w6140) -> ("error out"=w6156:errorcluster, "State Machine out"=w6159:refnum<class "State Machine.lvclass">)  [unwired: 7 in]
                n2857 = call-dynamic "Write State Machine.vi"("error in (no error)"=w6156, "State Machine.lvclass"=w6159, "Device in"=w6158) -> ("error out"=w6161:errorcluster, "Device out"=w6160:refnum<class "Channel.lvclass">)  [unwired: 7 in]
              }
            }
            n2858 = case shown="True" w5843 {
              tunnel: [w6112 w6136] -> w5951
              tunnel: [w6113 w6135] -> w5950
              tunnel: w5917 -> [w6113 w6130]
              tunnel: w5916 -> [w6112 w6129]
              frame False {
              }
              frame True {
                # "command WRITE_SETUP"
                # "command SET SUFFIX"
                n2859 = call-dynamic "Read State Machine.vi"("error in (no error)"=w6129, "Device in"=w6130) -> ("error out"=w6117:errorcluster, "State Machine.lvclass"=w6116:refnum<class "State Machine.lvclass">, "Device out"=w6133:refnum<class "Channel.lvclass">)  [unwired: 7 in]
